vi "HRR-UartConfig.vi"(8 "error in (no error)":errorcluster, 11 "VISA resource name in":refnum<visa-resource-name>="ASRL2::INSTR") -> (0 "error out":errorcluster, 3 "VISA resource name out":refnum<visa-resource-name>)   [LabVIEW 2019]
uses:
  <vilib>/myRIO/Instrument Drivers/Onboard IO/UART/typedef/VISA Configuration.ctl
  <vilib>/Instr/_visa.llb/VISA Configure Serial Port (Instr).vi
  <vilib>/myRIO/Instrument Drivers/Onboard IO/UART/UART.lvlib
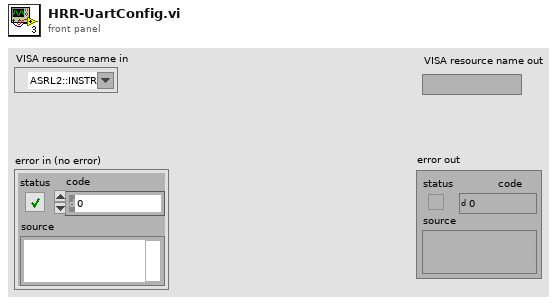
[diagram p1: front panel]
types:
  T1 = typedef "UART.lvlib/VISA Configuration.ctl" = cluster{"baud rate (9600)":u32, "data bits (8)":u16, "parity (0:none)":enum16{"None", "Odd", "Even", "Mark", "Space"}, "stop bits (10: 1 bit)":u16, "flow control (0:none)":u16, "termination char\n(0xA = '\\n' = LF) ":u8, "Enable Termination\nChar (T)":bool, "timeout (10sec)":u32}
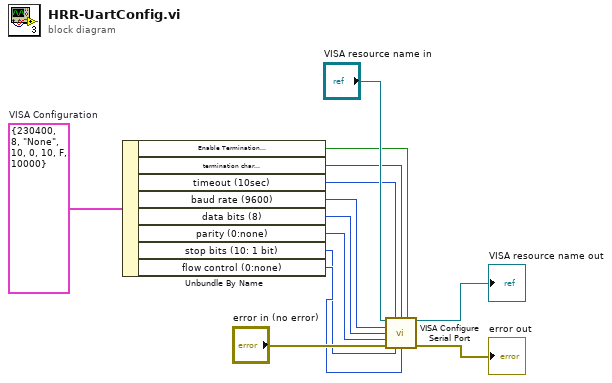
[diagram p0: block diagram]
diagram:
  w12 = T1 {"baud rate (9600)"=230400, "data bits (8)"=8, "parity (0:none)"=enum."None", "stop bits (10: 1 bit)"=10, "flow control (0:none)"=0, "termination char\n(0xA = '\\n' = LF) "=10, "Enable Termination\nChar (T)"=FALSE, "timeout (10sec)"=10000}  # VISA Configuration
  n1 = Unbundle By Name(w12) -> ("Enable Termination\nChar (T)"=w10:bool, "termination char\n(0xA = '\\n' = LF)"=w9:u8, "timeout (10sec)"=w8:u32, "baud rate (9600)"=w3:u32, "data bits (8)"=w4:u16, "parity (0:none)"=w5:enum16{"None", "Odd", "Even", "Mark", "Space"}, "stop bits (10: 1 bit)"=w6:u16, "flow control (0:none)"=w7:u16)
  n2 = call-poly "VISA Configure Serial Port"("VISA resource name"="VISA resource name in", "timeout (10sec)"=w8, "termination char\n(0xA = '\\n' = LF)"=w9, "Enable Termination\nChar (T)"=w10, "baud rate (9600)"=w3, "data bits (8)"=w4, "parity (0:none)"=w5, "error in (no error)"="error in (no error)", "stop bits (10: 1 bit)"=w6, "flow control (0:none)"=w7) -> ("VISA resource name out"=→"VISA resource name out":refnum<visa-resource-name>, "error out"=→"error out":errorcluster)  [unwired: 4 in]
